vi "addCore.vi"(8 "error in (no error)":errorcluster, 9 "Num2":dbl, 10 "Num1":dbl, 11 "Adder in":refnum<class "Adder.lvclass">) -> (0 "error out":errorcluster, 2 "Result":dbl, 3 "Adder out":refnum<class "Adder.lvclass">)   [LabVIEW 2018, in "extA.lvlib" / "Adder.lvclass"]
uses:
  Adder.lvclass
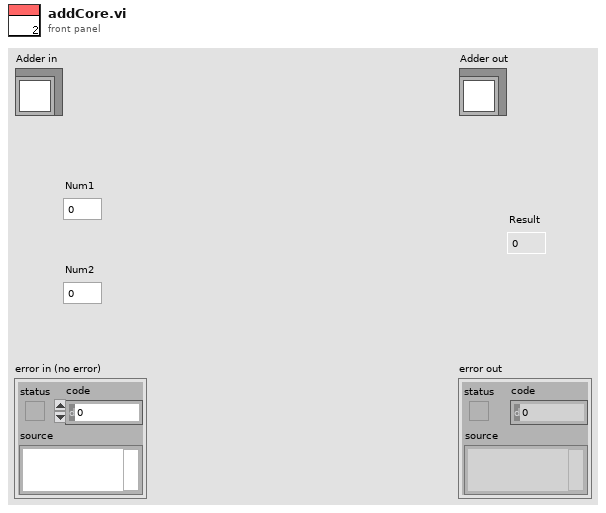
[diagram p1: front panel]
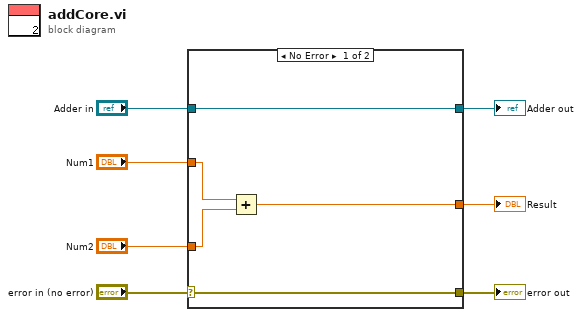
[diagram p0: block diagram]
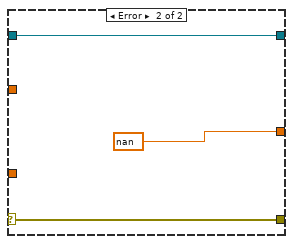
[diagram p2: hidden frame]
diagram:
  n1 = case shown="No Error" "error in (no error)" {
    selector: "error in (no error)" -> [w11 w15]
    tunnel: [w11 w15] -> w6
    tunnel: [w12 w14] -> w4
    tunnel: "Adder in" -> [w12 w14]
    tunnel: "Num1" -> [w10 _]
    tunnel: "Num2" -> [w9 _]
    tunnel: [w8 nan] -> w1
    frame No Error {
      n2 = Add(x=w10, y=w9) -> (x+y=w8:dbl)
    }
    frame Error {
    }
  }
  "error out" <- w6
  "Adder out" <- w4
  "Result" <- w1
